vi "set task timing.vi"(8 "error in (no error)":errorcluster, 11 "Waveform in":refnum<class "Waveform.lvclass">) -> (0 "error out":errorcluster, 3 "Waveform out":refnum<class "Waveform.lvclass">)   [LabVIEW 2012, in "Waveform.lvclass"]
uses:
  Waveform.lvclass
  Waveform.lvclass/Waveform.ctl
  <vilib>/DAQmx/configure/timing.llb/DAQmx Timing (Implicit).vi
  <vilib>/DAQmx/configure/timing.llb/DAQmx Timing (Sample Clock).vi
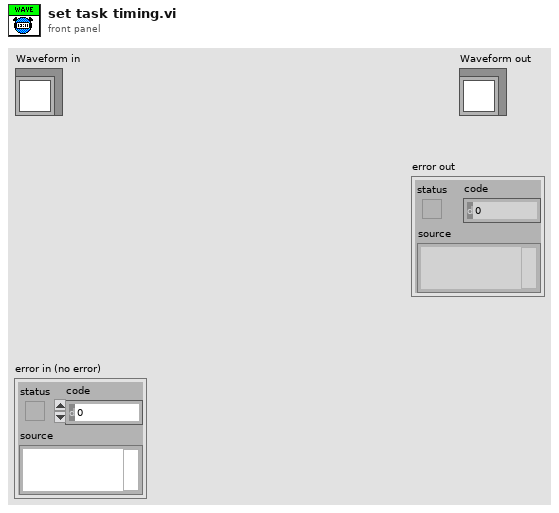
[diagram p1: front panel]
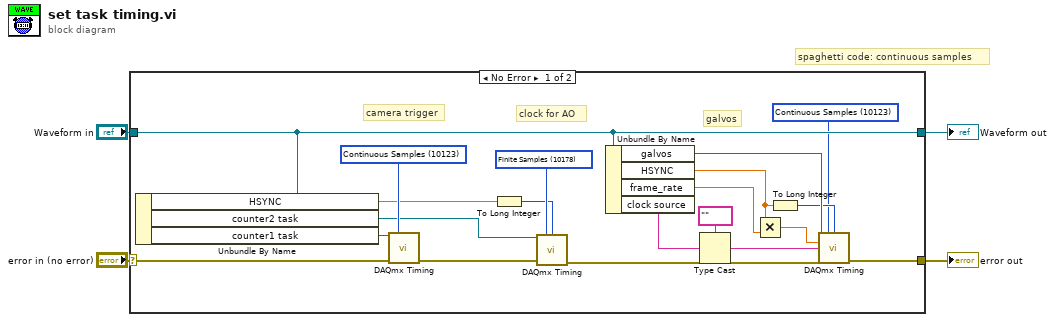
[diagram p0: block diagram]
diagram:
  # "spaghetti code: continuous samples"
  n1 = case shown="No Error" "error in (no error)" {
    selector: "error in (no error)" -> [w22 w26]
    tunnel: [w6 w26] -> w3
    tunnel: [w19 w25] -> w1
    tunnel: "Waveform in" -> [w19 w25]
    frame No Error {
      w12 = 10178 items=["Finite Samples"=10178, "Continuous Samples"=10123, "Hardware Timed Single Point"=12522] ("sample mode")
      w16 = 10123 items=["Finite Samples"=10178, "Continuous Samples"=10123, "Hardware Timed Single Point"=12522] ("sample mode")
      w24 = 10123 items=["Finite Samples"=10178, "Continuous Samples"=10123, "Hardware Timed Single Point"=12522] ("sample mode")
      # "galvos"
      # "camera trigger"
      # "clock for AO"
      n2 = Unbundle By Name(w19) -> ("HSYNC"=w10:dbl, "counter2 task"=w11:refnum<k21>, "counter1 task"=w23:refnum<k21>)
      n3 = call-poly <vilib>:"DAQmx Timing.vi"("task/channels in"=w23, "sample mode"=w24, "error in"=w22) -> ("error out"=w14:errorcluster)  [unwired: 11 in, 1 out]
      n4 = To Long Integer(number=w10) -> (32bit integer=w9:i32)
      n5 = call-poly <vilib>:"DAQmx Timing.vi"("task/channels in"=w11, "sample mode"=w12, "samples per channel"=w9, "error in"=w14) -> ("error out"=w13:errorcluster)  [unwired: 10 in, 1 out]
      n6 = Unbundle By Name(w19) -> ("galvos"=w18:refnum<k21>, "HSYNC"=w20:dbl, "frame_rate"=w21:dbl, "clock source"=w8:string)
      n7 = Type Cast(type=tag "" ("source"), x=w8) -> (*(type *) &x=w5:tag)
      n8 = Multiply(x=w20, y=w21) -> (x*y=w15:dbl)
      n9 = To Long Integer(number=w20) -> (32bit integer=w17:i32)
      n10 = call-poly <vilib>:"DAQmx Timing.vi"("task/channels in"=w18, "sample mode"=w16, "samples per channel"=w17, "rate"=w15, "source"=w5, "error in"=w13) -> ("error out"=w6:errorcluster)  [unwired: 8 in, 1 out]
    }
    frame Error {
    }
  }
  "error out" <- w3
  "Waveform out" <- w1
